vi "Filter.vi"(0 "parameter cluster":T2, 1 "Mode":T1, 5 "demand":dbl=1.0 format="%#_13g", 7 "max speed":dbl=1.0 format="%#_13g", 9 "dt":i32=1, 11 "error in":errorcluster, 12 "reset":bool) -> (6 "filtered signal":dbl format="%#_13g", 15 "error out":errorcluster)   [LabVIEW 2015]
uses:
  TypeDefs/Parameters.ctl
  TypeDefs/Modes.ctl
  RealTimeFilter.lvlib
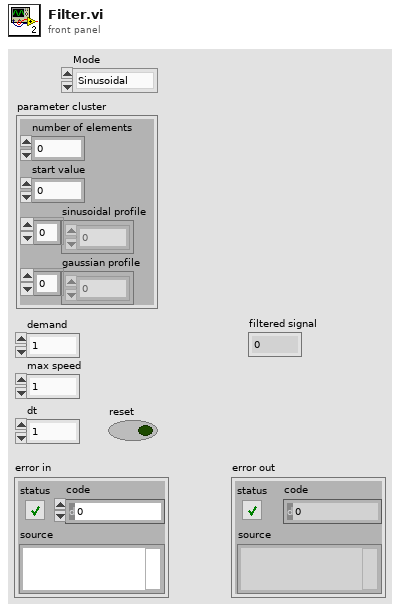
[diagram p1: front panel]
types:
  T1 = typedef "RealTimeFilter.lvlib/Modes.ctl" = enum16{"Sinusoidal", "Gaussian"}
  T2 = typedef "RealTimeFilter.lvlib/Parameters.ctl" = cluster{"number of elements":i32, "start value":dbl, "sinusoidal profile":dbl[], "gaussian profile":dbl[]}
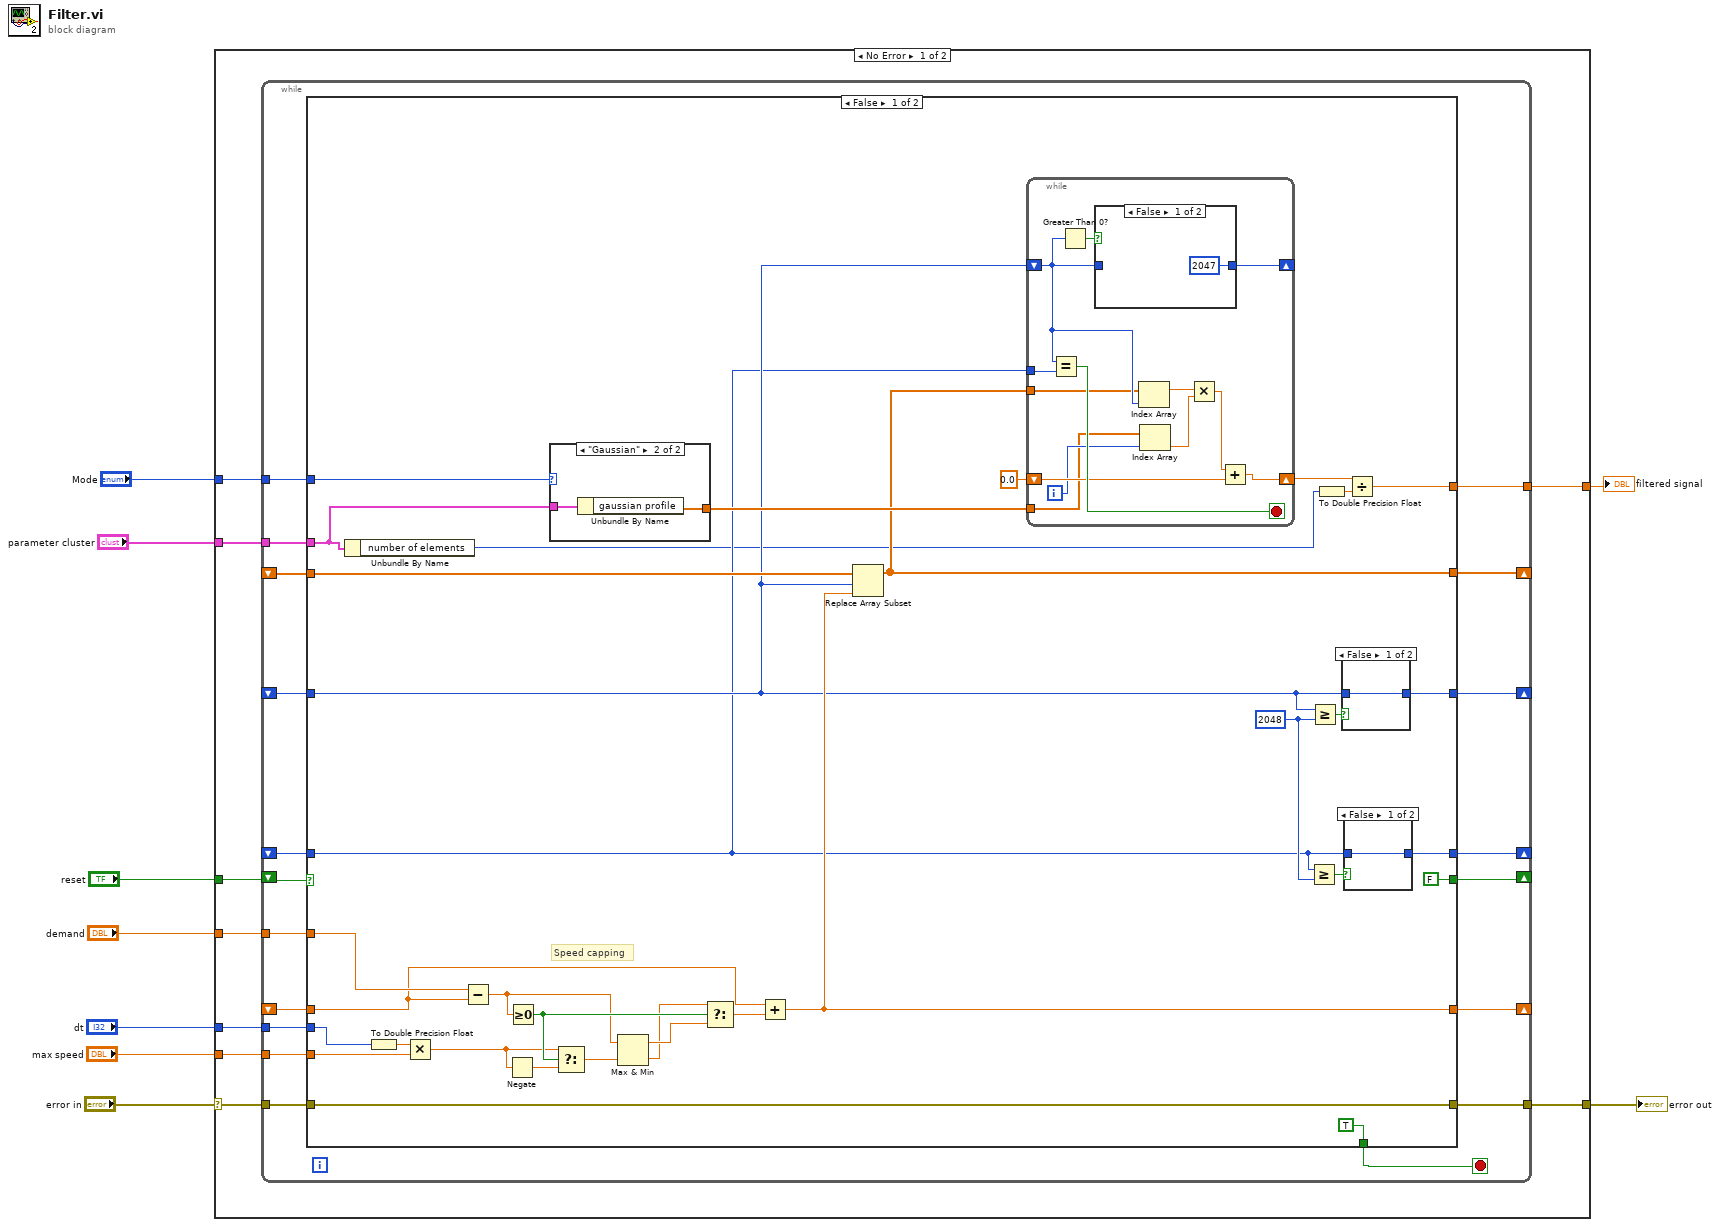
[diagram p0: block diagram]
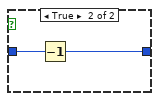
[diagram p2: hidden frame]
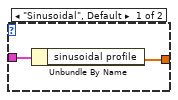
[diagram p3: hidden frame]
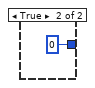
[diagram p4: hidden frame]
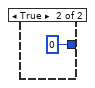
[diagram p5: hidden frame]
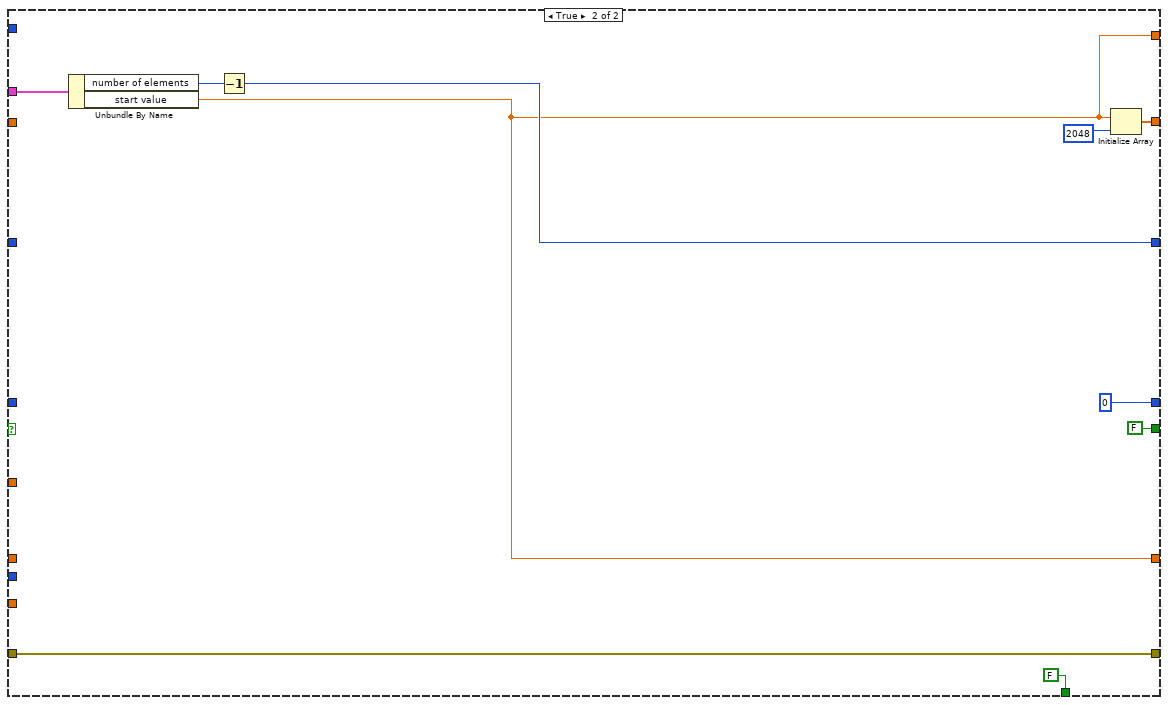
[diagram p6: hidden frame]
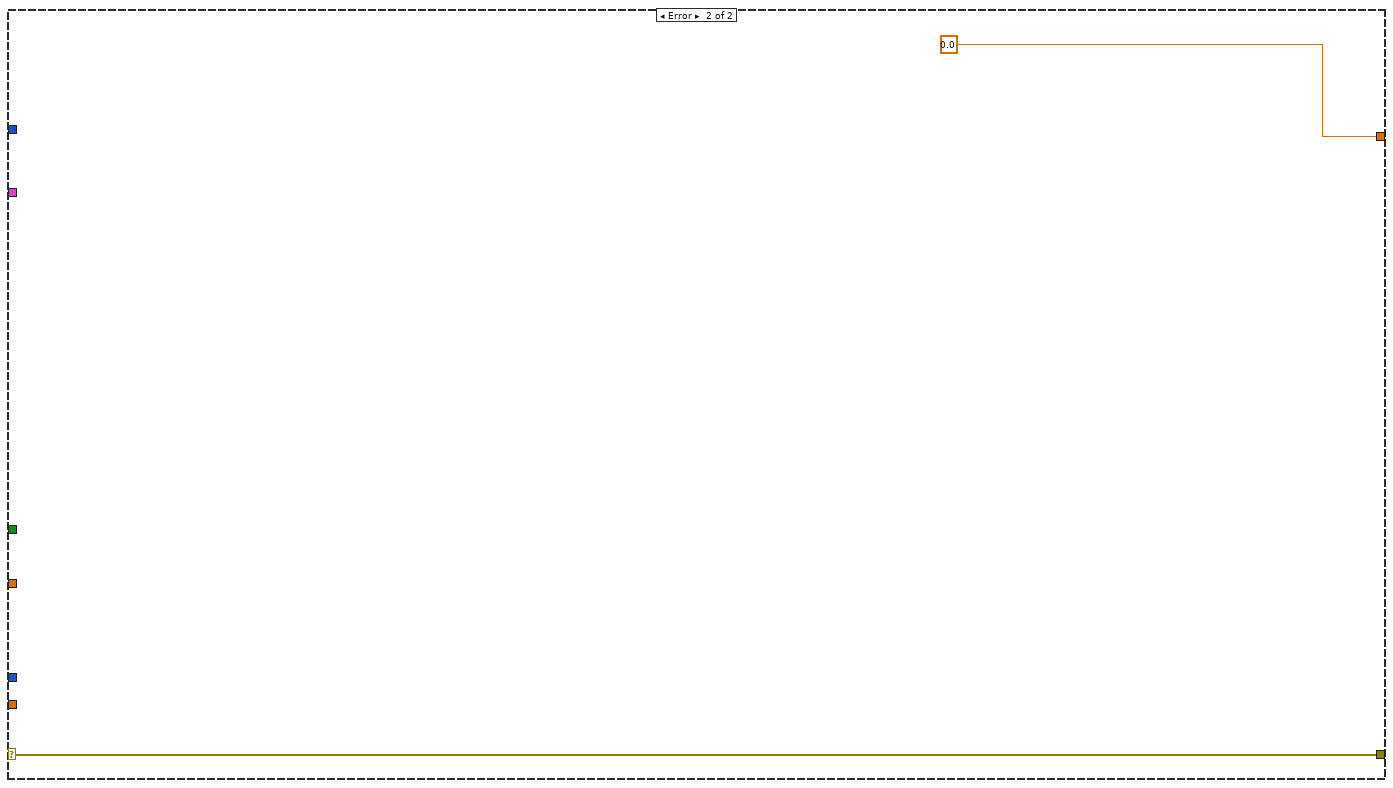
[diagram p7: hidden frame]
diagram:
  n1 = case shown="No Error" "error in" {
    selector: "error in" -> [w14 w107]
    tunnel: "demand" -> [w18 _]
    tunnel: "max speed" -> [w17 _]
    tunnel: "dt" -> [w16 _]
    tunnel: [w15 w107] -> w6
    tunnel: "reset" -> [w13 _]
    tunnel: [w10 0.0 ("filtered signal")] -> w3
    tunnel: "parameter cluster" -> [w12 _]
    tunnel: "Mode" -> [w11 _]
    frame No Error {
      n2 = while {
        tunnel: w18 -> [w35]
        tunnel: w17 -> [w37]
        tunnel: w16 -> [w36]
        shift-right: [w27] -> _
        shift-left: _ -> [w34]
        tunnel: [w25] -> w15
        tunnel: w14 -> [w24]
        shift-right: [w33] -> _
        shift-left: _ -> [w31]
        shift-right: [w32] -> _
        shift-left: _ -> [w30]
        tunnel: w12 -> [w29]
        tunnel: w11 -> [w28]
        shift-right: [w22] -> _
        shift-left: w13 -> [w26]
        shift-right: [w21] -> _
        shift-left: _ -> [w20]
        tunnel: [w19] -> w10
        stop <- w23 stop-if-true
        n3 = case shown="False" w26 {
          tunnel: w37 -> [w65 _]
          tunnel: w36 -> [w64 _]
          tunnel: w35 -> [w60 _]
          tunnel: w34 -> [w59 _]
          tunnel: [w58 w97] -> w33
          tunnel: [w57 0 ("t")] -> w32
          tunnel: w31 -> [w44 _]
          tunnel: w30 -> [w43 _]
          tunnel: w29 -> [w38 w104]
          tunnel: w28 -> [w56 _]
          tunnel: [w51 w96] -> w27
          tunnel: [w49 w103] -> w25
          tunnel: w24 -> [w49 w103]
          tunnel: [TRUE FALSE] -> w23
          tunnel: [FALSE FALSE] -> w22
          tunnel: [w46 w99] -> w21
          tunnel: w20 -> [w45 _]
          tunnel: [w39 w96] -> w19
          frame False {
            w53 = 2048
            # "Speed capping"
            n4 = Unbundle By Name(w38) -> ("number of elements"=w40:i32)
            n5 = To Double Precision Float(number=w64) -> (double precision float=w63:dbl)
            n6 = Multiply(x=w63, y=w65) -> (x*y=w62:dbl)
            n7 = Subtract(x=w60, y=w59) -> (x-y=w66:dbl)
            n8 = Negate(x=w62) -> (-x=w71:dbl)
            n9 = Greater Or Equal To 0?(x=w66) -> (x >= 0?=w69:bool)
            n10 = case shown="\"Gaussian\"" w56 {
              tunnel: [w88 w90] -> w52
              tunnel: w38 -> [w89 w91]
              frame "Sinusoidal", Default {
                n11 = Unbundle By Name(w89) -> ("sinusoidal profile"=w88:dbl[])
              }
              frame "Gaussian" {
                n12 = Unbundle By Name(w91) -> ("gaussian profile"=w90:dbl[])
              }
            }
            n13 = Select(t=w62, s=w69, f=w71) -> (s? t:f=w70:dbl)
            n14 = Max & Min(x=w66, y=w70) -> (max(x,y)=w68:dbl, min(x,y)=w67:dbl)
            n15 = Select(t=w67, s=w69, f=w68) -> (s? t:f=w61:dbl)
            n16 = Add(x=w59, y=w61) -> (x+y=w51:dbl)
            n17 = Replace Array Subset(array=w45, new element=w51, index=w44) -> (w46:dbl[])
            n18 = while {
              shift-right: [w83] -> _
              shift-left: w44 -> [w75]
              tunnel: w43 -> [w82]
              shift-right: [w78] -> w42
              shift-left: 0.0 -> [w80]
              tunnel: w52 -> [w74]
              tunnel: w46 -> [w72]
              i -> [w77]
              stop <- w81 stop-if-true
              n19 = Equal?(x=w75, y=w82) -> (x = y?=w81:bool)
              n20 = Greater Than 0?(x=w75) -> (x > 0?=w84:bool)
              n21 = case shown="False" w84 {
                tunnel: w75 -> [_ w87]
                tunnel: [2047 w86] -> w83
                frame False {
                }
                frame True {
                  n22 = Decrement(x=w87) -> (x-1=w86:i32)
                }
              }
              n23 = Index Array(array=w72, index=w75) -> (element=w76:dbl)
              n24 = Index Array(array=w74, index=w77) -> (element=w73:dbl)
              n25 = Multiply(x=w76, y=w73) -> (x*y=w79:dbl)
              n26 = Add(x=w79, y=w80) -> (x+y=w78:dbl)
            }
            n27 = Greater Or Equal?(x=w43, y=w53) -> (x >= y?=w55:bool)
            n28 = Greater Or Equal?(x=w44, y=w53) -> (x >= y?=w54:bool)
            n29 = To Double Precision Float(number=w40) -> (double precision float=w41:dbl)
            n30 = case shown="False" w54 {
              tunnel: w44 -> [w94 _]
              tunnel: [w94 0] -> w58
              frame False {
              }
              frame True {
              }
            }
            n31 = case shown="False" w55 {
              tunnel: [w92 0] -> w57
              tunnel: w43 -> [w92 _]
              frame False {
              }
              frame True {
              }
            }
            n32 = Divide(x=w42, y=w41) -> (x/y=w39:dbl)
          }
          frame True {
            n33 = Unbundle By Name(w104) -> ("number of elements"=w98:i32, "start value"=w96:dbl)
            n34 = Decrement(x=w98) -> (x-1=w97:i32)
            n35 = Initialize Array(w96, 2048) -> (w99:dbl[])
          }
        }
      }
    }
    frame Error {
    }
  }
  "filtered signal" <- w3
  "error out" <- w6
